vi "Destroy.vi"(8 "error in (no error)":errorcluster, 11 "List in":refnum<class "List.lvclass">) -> (0 "error out":errorcluster)   [LabVIEW 2017, in "LapDog.Collections.v0.Lists.lvlib" / "List.lvclass"]
doc: "Destroys the List object and releases all references used by the List Implementation object."
uses:
  List.lvclass
  List.lvclass/List.ctl
  ListImp/ListImp.lvclass
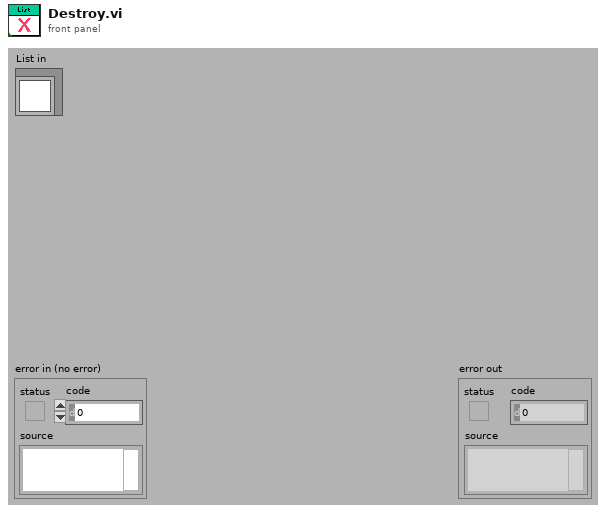
[diagram p1: front panel]
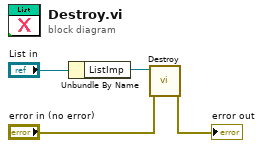
[diagram p0: block diagram]
diagram:
  n1 = Unbundle By Name("List in") -> ("ListImp"=w1:refnum<class "ListImp.lvclass">)
  n2 = call-dynamic "Destroy.vi"("error in (no error)"="error in (no error)", "ListImp in"=w1) -> ("error out"=→"error out":errorcluster)  [unwired: 9 in]
